vi "TOML to JSON.vi"(10 "Value":T2) -> (2 "JSON Value":T1)   [LabVIEW 2017]
uses:
  <vilib>/Erdos Miller/LV-JSON/JSON Value.ctl
  src/lib/TOML Key-Value Pair.ctl
  src/lib/TOML.lvlib
  src/lib/TOML Value.ctl
  <vilib>/Erdos Miller/LV-JSON/JSON Name-Value Pair.ctl
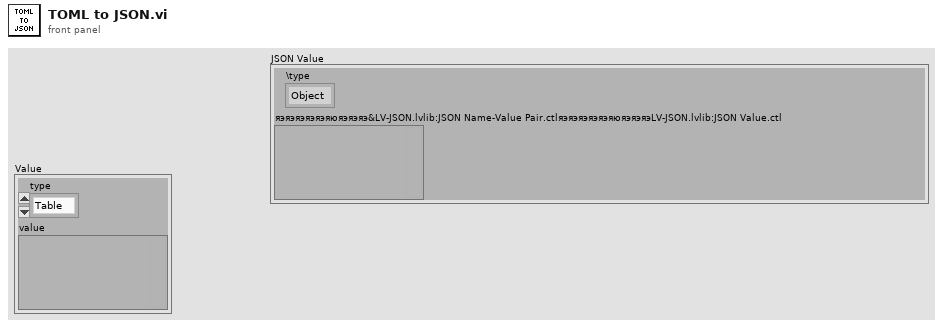
[diagram p1: front panel]
types:
  T1 = typedef "LV-JSON.lvlib/JSON Value.ctl" = cluster{"\\type":enum16{"Object", "Array", "String", "Number", "Boolean", "Null"}, "яэяэяэяэяэяюяэяэяэ&LV-JSON.lvlib:JSON Name-Value Pair.ctlяэяэяэяэяэяюяэяэяэLV-JSON.lvlib:JSON Value.ctl":variant}
  T2 = typedef "TOML.lvlib/TOML Value.ctl" = cluster{"type":enum16{"Table", "Array", "String", "Integer", "Float", "Boolean", "Offset Date-Time", "Local Date-Time", "Local Date", "Local Time"}, "value":variant}
  T3 = enum16{"Table", "Array", "String", "Integer", "Float", "Boolean", "Offset Date-Time", "Local Date-Time", "Local Date", "Local Time"}
  T4 = enum16{"Object", "Array", "String", "Number", "Boolean", "Null"}
  T5 = typedef "TOML.lvlib/TOML Key-Value Pair.ctl" = cluster{"Key":string, "Value":T2}
  T6 = typedef "LV-JSON.lvlib/JSON Name-Value Pair.ctl" = cluster{"Name":string, "Value":T1}
  T7 = cluster{"Type":enum16{"Table", "Array", "String", "Integer", "Float", "Boolean", "Offset Date-Time", "Local Date-Time", "Local Date", "Local Time"}, "value":variant}
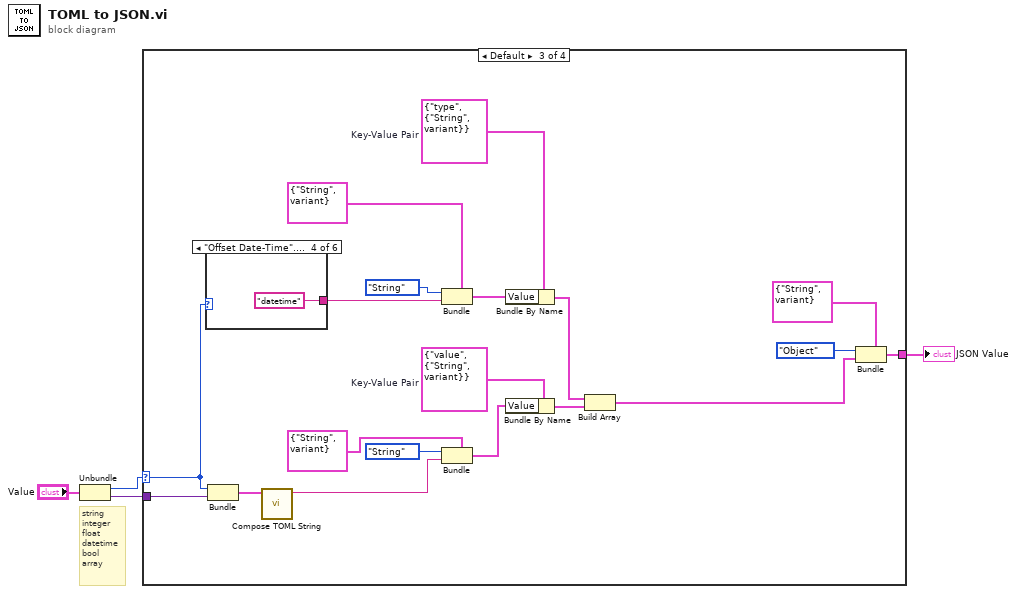
[diagram p0: block diagram]
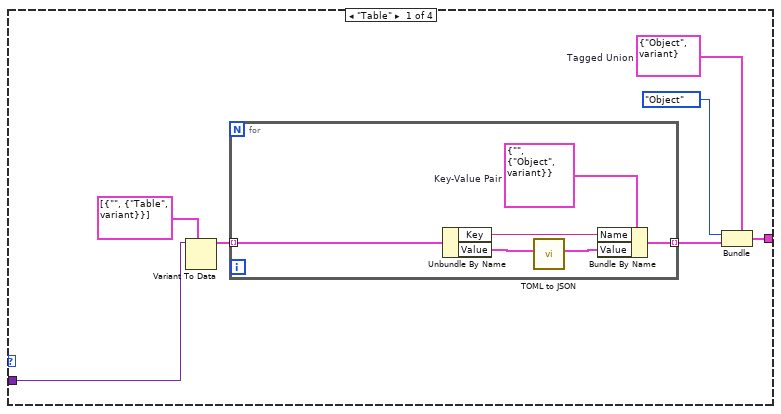
[diagram p2: hidden frame]
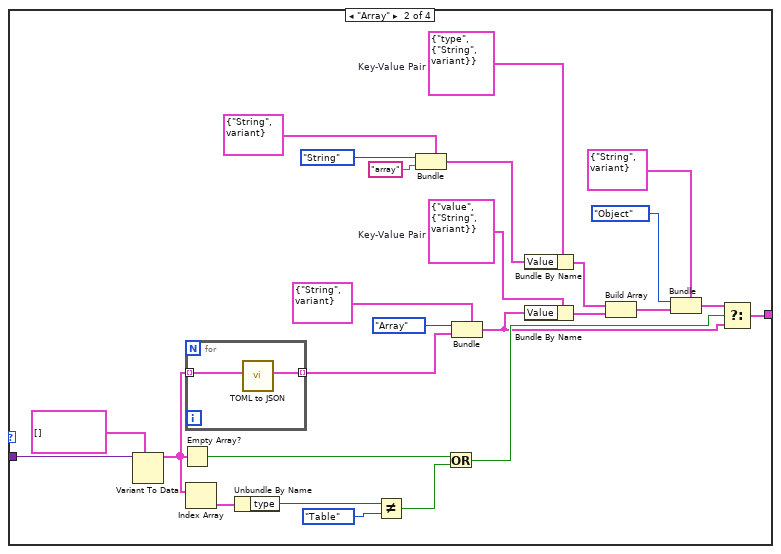
[diagram p3: hidden frame]
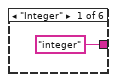
[diagram p4: hidden frame]
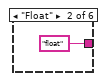
[diagram p5: hidden frame]
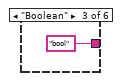
[diagram p6: hidden frame]
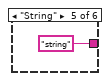
[diagram p7: hidden frame]
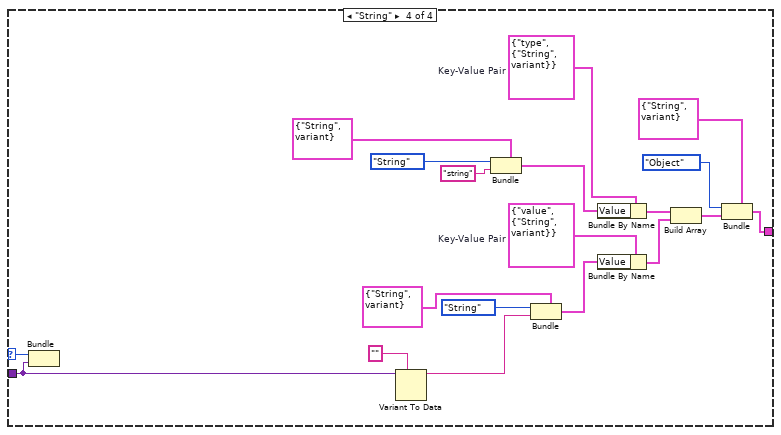
[diagram p9: hidden frame]
diagram:
  # "string\ninteger\nfloat\ndatetime\nbool\narray"
  n1 = Unbundle("Value") -> ("type"=w3:T3, "value"=w4:variant)
  n2 = case shown="Default" w3 {
    selector: w3 -> [_ _ w63 w88]
    tunnel: w4 -> [w11 w43 w64 w72]
    tunnel: [w7 w18 w50 w76] -> w1
    frame "Table" {
      w8 = T1 {"\\type"=enum."Object", "яэяэяэяэяэяюяэяэяэ&LV-JSON.lvlib:JSON Name-Value Pair.ctlяэяэяэяэяэяюяэяэяэLV-JSON.lvlib:JSON Value.ctl"=variant}  # Tagged Union
      n3 = Variant To Data(type=T5[] [{"Key"="", "Value"={"type"=enum."Table", "value"=variant}}], Variant=w11) -> (data=w9:T5[])  [unwired: 1 in, 1 out]
      n4 = for {
        tunnel: w9 -> [w17] mode=indexing
        tunnel: [w12] -> w5 mode=indexing
        w15 = T6 {"Name"="", "Value"={"\\type"=enum."Object", "яэяэяэяэяэяюяэяэяэ&LV-JSON.lvlib:JSON Name-Value Pair.ctlяэяэяэяэяэяюяэяэяэLV-JSON.lvlib:JSON Value.ctl"=variant}}  # Key-Value Pair
        n5 = Unbundle By Name(w17) -> ("Key"=w14:string, "Value"=w16:T2)
        n6 = call "TOML to JSON.vi"("Value"=w16) -> ("JSON Value"=w13:T1)  [unwired: 10 in]
        n7 = Bundle By Name(cluster=w15, "Name"=w14, "Value"=w13) -> (w12:T6)
      }
      n8 = Bundle(cluster=w8, "\\type"=T4."Object" ("\\type"), "яэяэяэяэяэяюяэяэяэ&LV-JSON.lvlib:JSON Name-Value Pair.ctlяэяэяэяэяэяюяэяэяэLV-JSON.lvlib:JSON Value.ctl"=w5) -> (w7:T1)
    }
    frame "Array" {
      w35 = T6 {"Name"="value", "Value"={"\\type"=enum."String", "яэяэяэяэяэяюяэяэяэ&LV-JSON.lvlib:JSON Name-Value Pair.ctlяэяэяэяэяэяюяэяэяэLV-JSON.lvlib:JSON Value.ctl"=variant}}  # Key-Value Pair
      w38 = T6 {"Name"="type", "Value"={"\\type"=enum."String", "яэяэяэяэяэяюяэяэяэ&LV-JSON.lvlib:JSON Name-Value Pair.ctlяэяэяэяэяэяюяэяэяэLV-JSON.lvlib:JSON Value.ctl"=variant}}  # Key-Value Pair
      n9 = Variant To Data(type=T2[] [], Variant=w43) -> (data=w26:T2[])  [unwired: 1 in, 1 out]
      n10 = Empty Array?(array=w26) -> (empty?=w22:bool)
      n11 = for {
        tunnel: w26 -> [w45] mode=indexing
        tunnel: [w44] -> w39 mode=indexing
        n12 = call "TOML to JSON.vi"("Value"=w45) -> ("JSON Value"=w44:T1)  [unwired: 10 in]
      }
      n13 = Index Array(array=w26) -> (element=w27:T2)  [unwired: 1 in]
      n14 = Unbundle By Name(w27) -> ("type"=w25:T3)
      n15 = Not Equal?(x=w25, y=T3."Table") -> (x != y?=w23:bool)
      n16 = Bundle(cluster=T1 {"\\type"=enum."String", "яэяэяэяэяэяюяэяэяэ&LV-JSON.lvlib:JSON Name-Value Pair.ctlяэяэяэяэяэяюяэяэяэLV-JSON.lvlib:JSON Value.ctl"=variant} ("Value"), "\\type"=T4."String" ("\\type"), "яэяэяэяэяэяюяэяэяэ&LV-JSON.lvlib:JSON Name-Value Pair.ctlяэяэяэяэяэяюяэяэяэLV-JSON.lvlib:JSON Value.ctl"="array") -> (w37:T1)
      n17 = Or(x=w22, y=w23) -> (x .or. y?=w21:bool)
      n18 = Bundle(cluster=T1 {"\\type"=enum."String", "яэяэяэяэяэяюяэяэяэ&LV-JSON.lvlib:JSON Name-Value Pair.ctlяэяэяэяэяэяюяэяэяэLV-JSON.lvlib:JSON Value.ctl"=variant} ("Value"), "\\type"=T4."Array" ("\\type"), "яэяэяэяэяэяюяэяэяэ&LV-JSON.lvlib:JSON Name-Value Pair.ctlяэяэяэяэяэяюяэяэяэLV-JSON.lvlib:JSON Value.ctl"=w39) -> (w19:T1)
      n19 = Bundle By Name(cluster=w38, "Value"=w37) -> (w33:T6)
      n20 = Bundle By Name(cluster=w35, "Value"=w19) -> (w32:T6)
      n21 = Build Array(w33, w32) -> (w31:T6[])
      n22 = Bundle(cluster=T1 {"\\type"=enum."String", "яэяэяэяэяэяюяэяэяэ&LV-JSON.lvlib:JSON Name-Value Pair.ctlяэяэяэяэяэяюяэяэяэLV-JSON.lvlib:JSON Value.ctl"=variant} ("Value"), "\\type"=T4."Object" ("\\type"), "яэяэяэяэяэяюяэяэяэ&LV-JSON.lvlib:JSON Name-Value Pair.ctlяэяэяэяэяэяюяэяэяэLV-JSON.lvlib:JSON Value.ctl"=w31) -> (w20:T1)
      n23 = Select(t=w20, s=w21, f=w19) -> (s? t:f=w18:T1)
    }
    frame Default {
      w55 = T6 {"Name"="value", "Value"={"\\type"=enum."String", "яэяэяэяэяэяюяэяэяэ&LV-JSON.lvlib:JSON Name-Value Pair.ctlяэяэяэяэяэяюяэяэяэLV-JSON.lvlib:JSON Value.ctl"=variant}}  # Key-Value Pair
      w61 = T6 {"Name"="type", "Value"={"\\type"=enum."String", "яэяэяэяэяэяюяэяэяэ&LV-JSON.lvlib:JSON Name-Value Pair.ctlяэяэяэяэяэяюяэяэяэLV-JSON.lvlib:JSON Value.ctl"=variant}}  # Key-Value Pair
      n24 = case shown="\"Offset Date-Time\"..\"Local Time\"" w63 {
        tunnel: ["integer" "float" "bool" "datetime" "string" _] -> w49
        frame "Integer" {
        }
        frame "Float" {
        }
        frame "Boolean" {
        }
        frame "Offset Date-Time".."Local Time" {
        }
        frame "String" {
        }
        frame Default {
        }
      }
      n25 = Bundle("Type"=w63, "value"=w64) -> (w62:T7)  [unwired: 1 in]
      n26 = call "Compose TOML String.vi"("Value"=w62) -> ("String"=w48:string)  [unwired: 9 in, 1 out]
      n27 = Bundle(cluster=T1 {"\\type"=enum."String", "яэяэяэяэяэяюяэяэяэ&LV-JSON.lvlib:JSON Name-Value Pair.ctlяэяэяэяэяэяюяэяэяэLV-JSON.lvlib:JSON Value.ctl"=variant} ("Value"), "\\type"=T4."String" ("\\type"), "яэяэяэяэяэяюяэяэяэ&LV-JSON.lvlib:JSON Name-Value Pair.ctlяэяэяэяэяэяюяэяэяэLV-JSON.lvlib:JSON Value.ctl"=w49) -> (w60:T1)
      n28 = Bundle(cluster=T1 {"\\type"=enum."String", "яэяэяэяэяэяюяэяэяэ&LV-JSON.lvlib:JSON Name-Value Pair.ctlяэяэяэяэяэяюяэяэяэLV-JSON.lvlib:JSON Value.ctl"=variant} ("Value"), "\\type"=T4."String" ("\\type"), "яэяэяэяэяэяюяэяэяэ&LV-JSON.lvlib:JSON Name-Value Pair.ctlяэяэяэяэяэяюяэяэяэLV-JSON.lvlib:JSON Value.ctl"=w48) -> (w56:T1)
      n29 = Bundle By Name(cluster=w61, "Value"=w60) -> (w53:T6)
      n30 = Bundle By Name(cluster=w55, "Value"=w56) -> (w52:T6)
      n31 = Build Array(w53, w52) -> (w51:T6[])
      n32 = Bundle(cluster=T1 {"\\type"=enum."String", "яэяэяэяэяэяюяэяэяэ&LV-JSON.lvlib:JSON Name-Value Pair.ctlяэяэяэяэяэяюяэяэяэLV-JSON.lvlib:JSON Value.ctl"=variant} ("Value"), "\\type"=T4."Object" ("\\type"), "яэяэяэяэяэяюяэяэяэ&LV-JSON.lvlib:JSON Name-Value Pair.ctlяэяэяэяэяэяюяэяэяэLV-JSON.lvlib:JSON Value.ctl"=w51) -> (w50:T1)
    }
    frame "String" {
      w81 = T6 {"Name"="value", "Value"={"\\type"=enum."String", "яэяэяэяэяэяюяэяэяэ&LV-JSON.lvlib:JSON Name-Value Pair.ctlяэяэяэяэяэяюяэяэяэLV-JSON.lvlib:JSON Value.ctl"=variant}}  # Key-Value Pair
      w87 = T6 {"Name"="type", "Value"={"\\type"=enum."String", "яэяэяэяэяэяюяэяэяэ&LV-JSON.lvlib:JSON Name-Value Pair.ctlяэяэяэяэяэяюяэяэяэLV-JSON.lvlib:JSON Value.ctl"=variant}}  # Key-Value Pair
      n33 = Bundle("Type"=w88, "value"=w72) -> ()  [unwired: 1 in, 1 out]
      n34 = Variant To Data(type="", Variant=w72) -> (data=w70:string)  [unwired: 1 in, 1 out]
      n35 = Bundle(cluster=T1 {"\\type"=enum."String", "яэяэяэяэяэяюяэяэяэ&LV-JSON.lvlib:JSON Name-Value Pair.ctlяэяэяэяэяэяюяэяэяэLV-JSON.lvlib:JSON Value.ctl"=variant} ("Value"), "\\type"=T4."String" ("\\type"), "яэяэяэяэяэяюяэяэяэ&LV-JSON.lvlib:JSON Name-Value Pair.ctlяэяэяэяэяэяюяэяэяэLV-JSON.lvlib:JSON Value.ctl"="string") -> (w86:T1)
      n36 = Bundle(cluster=T1 {"\\type"=enum."String", "яэяэяэяэяэяюяэяэяэ&LV-JSON.lvlib:JSON Name-Value Pair.ctlяэяэяэяэяэяюяэяэяэLV-JSON.lvlib:JSON Value.ctl"=variant} ("Value"), "\\type"=T4."String" ("\\type"), "яэяэяэяэяэяюяэяэяэ&LV-JSON.lvlib:JSON Name-Value Pair.ctlяэяэяэяэяэяюяэяэяэLV-JSON.lvlib:JSON Value.ctl"=w70) -> (w82:T1)
      n37 = Bundle By Name(cluster=w87, "Value"=w86) -> (w79:T6)
      n38 = Bundle By Name(cluster=w81, "Value"=w82) -> (w78:T6)
      n39 = Build Array(w79, w78) -> (w77:T6[])
      n40 = Bundle(cluster=T1 {"\\type"=enum."String", "яэяэяэяэяэяюяэяэяэ&LV-JSON.lvlib:JSON Name-Value Pair.ctlяэяэяэяэяэяюяэяэяэLV-JSON.lvlib:JSON Value.ctl"=variant} ("Value"), "\\type"=T4."Object" ("\\type"), "яэяэяэяэяэяюяэяэяэ&LV-JSON.lvlib:JSON Name-Value Pair.ctlяэяэяэяэяэяюяэяэяэLV-JSON.lvlib:JSON Value.ctl"=w77) -> (w76:T1)
    }
  }
  "JSON Value" <- w1
